vi "M9700 Modbus Demo.vi"() -> ()   [LabVIEW 2018]
uses:
  M9700 Driver/86/vi.lib/M9700 Modbus.llb/CTL CMD Register.ctl
  M9700 Driver/86/vi.lib/M9700 Modbus.llb/CTL Register Address.ctl
  <vilib>/Instr/_visa.llb/VISA Configure Serial Port (Instr).vi
panel:
  in  "Configure Serial Port":bool
  in  "error in (no error)":errorcluster
  out "error out":errorcluster
  in  "Short Mode":bool
  in  "Set Power":bool
  in  "Set Resistance":bool
  in  "Set Current":bool
  in  "Set Voltage":bool
  in  "Power(W)":sgl=30.0 format="%#.5g"
  in  "Resistance(Ohm)":sgl=100.0 format="%#.5g"
  in  "Current(A)":sgl=1.0 format="%#.5g"
  in  "Voltage(V)":sgl=10.0 format="%#.5g"
  out "Actual Power(W)":sgl format="%#.5g"
  out "Actual Resistance(Ohm)":sgl format="%#.5g"
  out "Actual Current(A)":sgl format="%#.5g"
  out "Actual Voltage(V)":sgl format="%#.5g"
  in  "Read Actual Value":bool
  in  "Input OFF":bool
  in  "Input ON":bool
  out "Input State":bool
  in  "Read Input State":bool
  in  "Load Address":u8=1 min=1 max=200 format="%.0x"
  in  "Serial Port:":refnum<visa-resource-name>="COM1"
  in  "About":bool
  in  "Exit":bool
  in  "Parity:":u16(ring) items=["  None", "  Odd", "  Even"]
  in  "BaudRate:":u16(ring)=1 items=["  2400", "  9600", "  14400", "  28800", "  57600", "  115200"]
  # "This example shows how communication is generated between M97 series electronic load \n and LabVIEW Program by M9700 MODBUS LabVIEW Driver. \n."
  # "Serial Port Parameter:"
  # "Work Mode:"
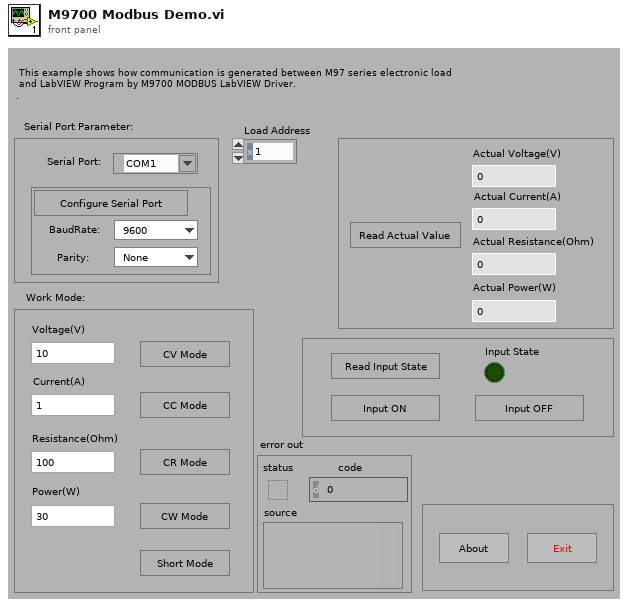
[diagram p1: front panel]
types:
  T1 = typedef "CTL CMD Register.ctl" = u8
  T2 = typedef "CTL Register Address.ctl" = u16
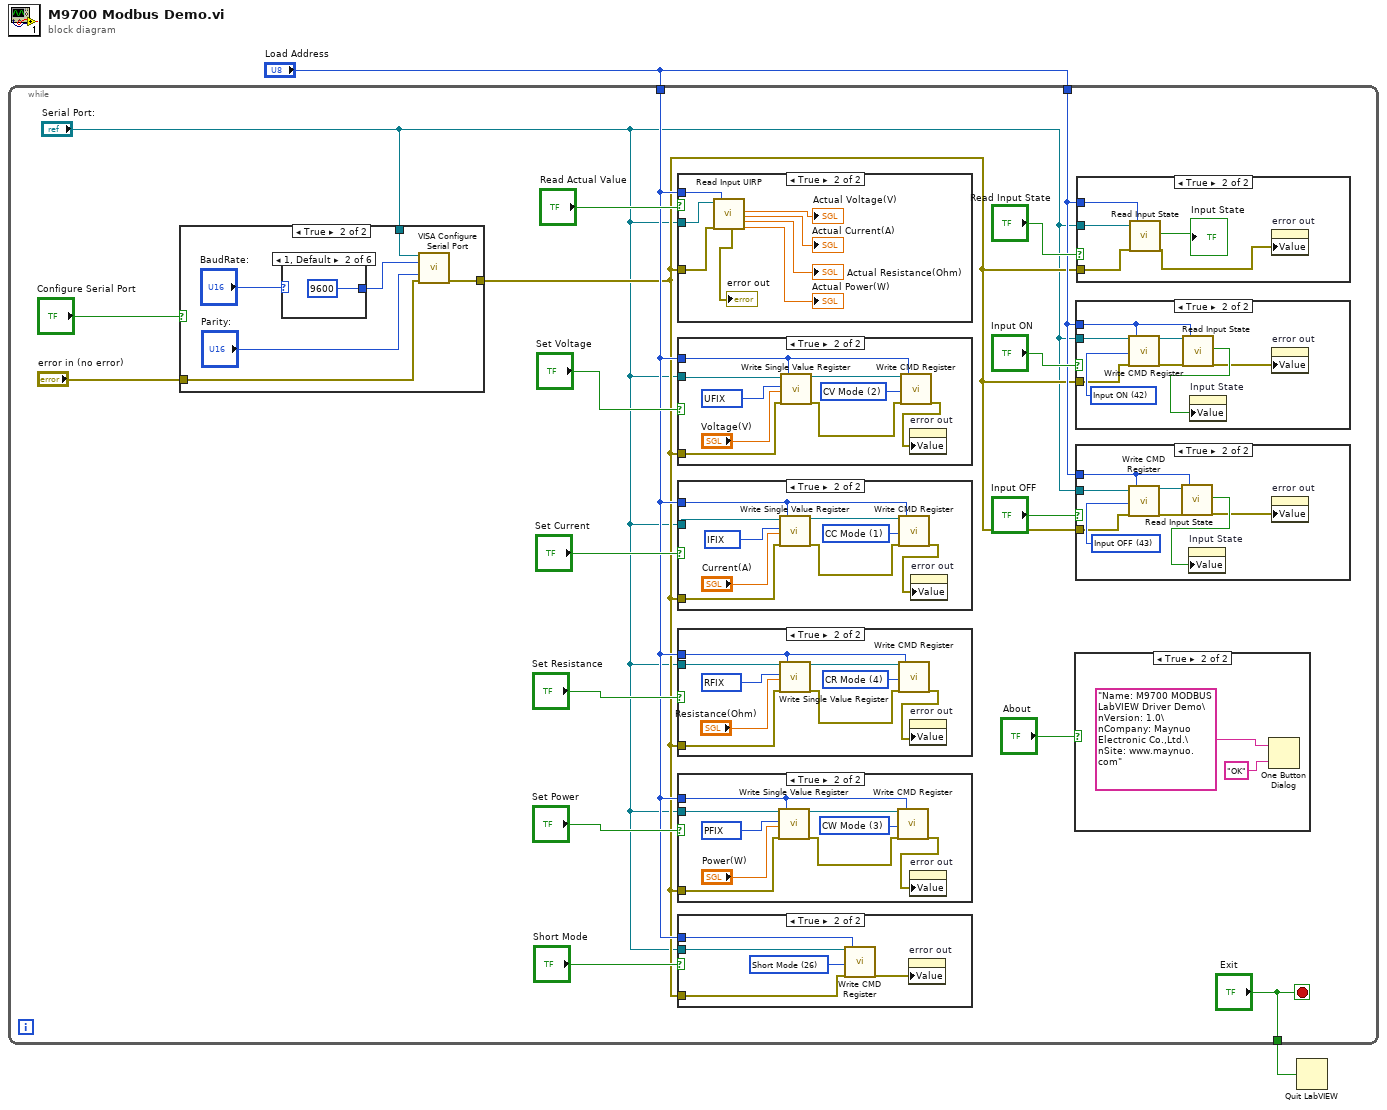
[diagram p0: block diagram]
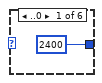
[diagram p3: hidden frame]
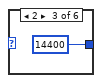
[diagram p4: hidden frame]
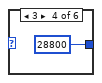
[diagram p5: hidden frame]
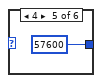
[diagram p6: hidden frame]
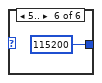
[diagram p7: hidden frame]
diagram:
  n1 = while {
    tunnel: ["Exit"] -> w2
    tunnel: "Load Address" -> [w12]
    tunnel: "Load Address" -> [w8]
    stop <- "Exit" stop-if-true
    n2 = case shown="True" "Configure Serial Port" {
      tunnel: [w20 w26] -> w6
      tunnel: "Serial Port:" -> [_ w22]
      tunnel: "error in (no error)" -> [w20 w21]
      frame False {
      }
      frame True {
        n3 = case shown="1, Default" "BaudRate:" {
          tunnel: [2400 9600 14400 28800 57600 115200] -> w24
          frame ..0 {
          }
          frame 1, Default {
          }
          frame 2 {
          }
          frame 3 {
          }
          frame 4 {
          }
          frame 5.. {
          }
        }
        n4 = call-poly "VISA Configure Serial Port"("VISA resource name"=w22, "baud rate (9600)"=w24, "parity (0:none)"="Parity:", "error in (no error)"=w21) -> ("error out"=w26:errorcluster)  [unwired: 2 in, 9 out]
      }
    }
    n5 = case shown="True" "Read Actual Value" {
      tunnel: w12 -> [_ w104]
      tunnel: "Serial Port:" -> [_ w103]
      tunnel: w6 -> [_ w98]
      frame False {
      }
      frame True {
        n6 = call "Read Input UIRP.vi"("VISA resource name"=w103, "error in"=w98, "Load Address"=w104) -> ("error out"=→"error out":errorcluster, "Actual Voltage(V)"=→"Actual Voltage(V)":sgl, "Actual Current(A)"=→"Actual Current(A)":sgl, "Actual Resistance(Ohm)"=→"Actual Resistance(Ohm)":sgl, "Actual Power(W)"=→"Actual Power(W)":sgl)  [unwired: 12 out]
      }
    }
    n7 = case shown="True" "Set Voltage" {
      tunnel: w12 -> [_ w92]
      tunnel: "Serial Port:" -> [_ w96]
      tunnel: w6 -> [_ w90]
      frame False {
      }
      frame True {
        w91 = T1 2 items=["CC Mode"=1, "CV Mode"=2, "CW Mode"=3, "CR Mode"=4, "Short Mode"=26, "Set SysPara"=41, "Input ON"=42, "Input OFF"=43] ("CMD Register Value")
        w94 = T2 2563 items=["REMOTE"=1283, "ISTATE"=1296, "CMD"=2560, "IFIX"=2561, "UFIX"=2563, "PFIX"=2565, "RFIX"=2567, "IMAX"=2612, "UMAX"=2614, "PMAX"=2616, "U"=2816, "I"=2818, "MODEL"=2822, "EDITION"=2823] ("Register Address")
        n8 = call "Write Single Value Register.vi"("VISA resource name"=w96, "Starting Address(HEX)"=w94, "Register Single Value"="Voltage(V)", "error in"=w90, "Load Address"=w92) -> ("VISA resource name out"=w93:refnum<visa-resource-name>, "error out"=w89:errorcluster)  [unwired: 13 out]
        n9 = call "Write CMD Register.vi"("VISA resource name"=w93, "CMD Value"=w91, "error in"=w89, "Load Address"=w92) -> ("error out"=w88:errorcluster)  [unwired: 15 out]
        n10 = property on="error out" class="Clust (strict)"("Value"=w88) -> ()  [unwired: 2 in, 2 out]
      }
    }
    n11 = case shown="True" "Set Current" {
      tunnel: w12 -> [_ w87]
      tunnel: "Serial Port:" -> [_ w83]
      tunnel: w6 -> [_ w81]
      frame False {
      }
      frame True {
        w84 = T1 1 items=["CC Mode"=1, "CV Mode"=2, "CW Mode"=3, "CR Mode"=4, "Short Mode"=26, "Set SysPara"=41, "Input ON"=42, "Input OFF"=43] ("CMD Register Value")
        w86 = T2 2561 items=["REMOTE"=1283, "ISTATE"=1296, "CMD"=2560, "IFIX"=2561, "UFIX"=2563, "PFIX"=2565, "RFIX"=2567, "IMAX"=2612, "UMAX"=2614, "PMAX"=2616, "U"=2816, "I"=2818, "MODEL"=2822, "EDITION"=2823] ("Register Address")
        n12 = call "Write Single Value Register.vi"("VISA resource name"=w83, "Starting Address(HEX)"=w86, "Register Single Value"="Current(A)", "error in"=w81, "Load Address"=w87) -> ("VISA resource name out"=w82:refnum<visa-resource-name>, "error out"=w80:errorcluster)  [unwired: 13 out]
        n13 = call "Write CMD Register.vi"("VISA resource name"=w82, "CMD Value"=w84, "error in"=w80, "Load Address"=w87) -> ("error out"=w79:errorcluster)  [unwired: 15 out]
        n14 = property on="error out" class="Clust (strict)"("Value"=w79) -> ()  [unwired: 2 in, 2 out]
      }
    }
    n15 = case shown="True" "Set Resistance" {
      tunnel: "Serial Port:" -> [_ w76]
      tunnel: w12 -> [_ w78]
      tunnel: w6 -> [_ w72]
      frame False {
      }
      frame True {
        w73 = T1 4 items=["CC Mode"=1, "CV Mode"=2, "CW Mode"=3, "CR Mode"=4, "Short Mode"=26, "Set SysPara"=41, "Input ON"=42, "Input OFF"=43] ("CMD Register Value")
        w75 = T2 2567 items=["REMOTE"=1283, "ISTATE"=1296, "CMD"=2560, "IFIX"=2561, "UFIX"=2563, "PFIX"=2565, "RFIX"=2567, "IMAX"=2612, "UMAX"=2614, "PMAX"=2616, "U"=2816, "I"=2818, "MODEL"=2822, "EDITION"=2823] ("Register Address")
        n16 = call "Write Single Value Register.vi"("VISA resource name"=w76, "Starting Address(HEX)"=w75, "Register Single Value"="Resistance(Ohm)", "error in"=w72, "Load Address"=w78) -> ("VISA resource name out"=w77:refnum<visa-resource-name>, "error out"=w71:errorcluster)  [unwired: 13 out]
        n17 = call "Write CMD Register.vi"("VISA resource name"=w77, "CMD Value"=w73, "error in"=w71, "Load Address"=w78) -> ("error out"=w70:errorcluster)  [unwired: 15 out]
        n18 = property on="error out" class="Clust (strict)"("Value"=w70) -> ()  [unwired: 2 in, 2 out]
      }
    }
    n19 = case shown="True" "Set Power" {
      tunnel: "Serial Port:" -> [_ w69]
      tunnel: w12 -> [_ w67]
      tunnel: w6 -> [_ w64]
      frame False {
      }
      frame True {
        w65 = T1 3 items=["CC Mode"=1, "CV Mode"=2, "CW Mode"=3, "CR Mode"=4, "Short Mode"=26, "Set SysPara"=41, "Input ON"=42, "Input OFF"=43] ("CMD Register Value")
        w66 = T2 2565 items=["REMOTE"=1283, "ISTATE"=1296, "CMD"=2560, "IFIX"=2561, "UFIX"=2563, "PFIX"=2565, "RFIX"=2567, "IMAX"=2612, "UMAX"=2614, "PMAX"=2616, "U"=2816, "I"=2818, "MODEL"=2822, "EDITION"=2823] ("Register Address")
        n20 = call "Write Single Value Register.vi"("VISA resource name"=w69, "Starting Address(HEX)"=w66, "Register Single Value"="Power(W)", "error in"=w64, "Load Address"=w67) -> ("VISA resource name out"=w68:refnum<visa-resource-name>, "error out"=w62:errorcluster)  [unwired: 13 out]
        n21 = call "Write CMD Register.vi"("VISA resource name"=w68, "CMD Value"=w65, "error in"=w62, "Load Address"=w67) -> ("error out"=w61:errorcluster)  [unwired: 15 out]
        n22 = property on="error out" class="Clust (strict)"("Value"=w61) -> ()  [unwired: 2 in, 2 out]
      }
    }
    n23 = case shown="True" "Short Mode" {
      tunnel: "Serial Port:" -> [_ w60]
      tunnel: w12 -> [_ w58]
      tunnel: w6 -> [_ w57]
      frame False {
      }
      frame True {
        w59 = T1 26 items=["CC Mode"=1, "CV Mode"=2, "CW Mode"=3, "CR Mode"=4, "Short Mode"=26, "Set SysPara"=41, "Input ON"=42, "Input OFF"=43] ("CMD Register Value")
        n24 = call "Write CMD Register.vi"("VISA resource name"=w60, "CMD Value"=w59, "error in"=w57, "Load Address"=w58) -> ("error out"=w56:errorcluster)  [unwired: 15 out]
        n25 = property on="error out" class="Clust (strict)"("Value"=w56) -> ()  [unwired: 2 in, 2 out]
      }
    }
    n26 = case shown="True" "About" {
      frame False {
      }
      frame True {
        n27 = One Button Dialog(message="Name: M9700 MODBUS LabVIEW Driver Demo\nVersion: 1.0\nCompany: Maynuo Electronic Co.,Ltd.\nSite: www.maynuo.com", button name ("OK")="OK") -> ()  [unwired: 1 out]
      }
    }
    n28 = case shown="True" "Input ON" {
      tunnel: "Serial Port:" -> [_ w50]
      tunnel: w8 -> [_ w46]
      tunnel: w6 -> [_ w45]
      frame False {
      }
      frame True {
        w49 = T1 42 items=["CC Mode"=1, "CV Mode"=2, "CW Mode"=3, "CR Mode"=4, "Short Mode"=26, "Set SysPara"=41, "Input ON"=42, "Input OFF"=43] ("CMD Register Value")
        n29 = call "Write CMD Register.vi"("VISA resource name"=w50, "CMD Value"=w49, "error in"=w45, "Load Address"=w46) -> ("VISA resource name out"=w48:refnum<visa-resource-name>, "error out"=w44:errorcluster)  [unwired: 14 out]
        n30 = call "Read Input State.vi"("VISA resource name"=w48, "error in"=w44, "Load Address"=w46) -> ("Input State(ON/OFF)"=w47:bool, "error out"=w43:errorcluster)  [unwired: 15 out]
        n31 = property on="Input State" class="Bool (strict)"("Value"=w47) -> ()  [unwired: 2 in, 2 out]
        n32 = property on="error out" class="Clust (strict)"("Value"=w43) -> ()  [unwired: 2 in, 2 out]
      }
    }
    n33 = case shown="True" "Input OFF" {
      tunnel: "Serial Port:" -> [_ w42]
      tunnel: w8 -> [_ w39]
      tunnel: w6 -> [_ w37]
      frame False {
      }
      frame True {
        w41 = T1 43 items=["CC Mode"=1, "CV Mode"=2, "CW Mode"=3, "CR Mode"=4, "Short Mode"=26, "Set SysPara"=41, "Input ON"=42, "Input OFF"=43] ("CMD Register Value")
        n34 = call "Write CMD Register.vi"("VISA resource name"=w42, "CMD Value"=w41, "error in"=w37, "Load Address"=w39) -> ("VISA resource name out"=w40:refnum<visa-resource-name>, "error out"=w36:errorcluster)  [unwired: 14 out]
        n35 = call "Read Input State.vi"("VISA resource name"=w40, "error in"=w36, "Load Address"=w39) -> ("Input State(ON/OFF)"=w38:bool, "error out"=w35:errorcluster)  [unwired: 15 out]
        n36 = property on="Input State" class="Bool (strict)"("Value"=w38) -> ()  [unwired: 2 in, 2 out]
        n37 = property on="error out" class="Clust (strict)"("Value"=w35) -> ()  [unwired: 2 in, 2 out]
      }
    }
    n38 = case shown="True" "Read Input State" {
      tunnel: w8 -> [_ w55]
      tunnel: "Serial Port:" -> [_ w53]
      tunnel: w6 -> [_ w52]
      frame False {
      }
      frame True {
        n39 = call "Read Input State.vi"("VISA resource name"=w53, "error in"=w52, "Load Address"=w55) -> ("Input State(ON/OFF)"=→"Input State":bool, "error out"=w51:errorcluster)  [unwired: 15 out]
        n40 = property on="error out" class="Clust (strict)"("Value"=w51) -> ()  [unwired: 2 in, 2 out]
      }
    }
  }
  n41 = Quit LabVIEW(quit? (T)=w2) -> ()
